vi "calcDemandedPressureOutput.vi"(8 "error in (no error)":errorcluster, 9 "loopPeriod":dbl[unit]=5000.0 min=10.0 max=5000.0, 10 "Pressure Valve Opening (%)":dbl=2.0 min=1.0 max=4.0, 11 "SystemController in":refnum<class "SystemController.lvclass">) -> (0 "error out":errorcluster, 2 "rampOutput (%)":dbl=5000.0 min=10.0 max=5000.0, 3 "SystemController out":refnum<class "SystemController.lvclass">)   [LabVIEW 2015, in "SystemController.lvclass"]
uses:
  SystemController.lvclass
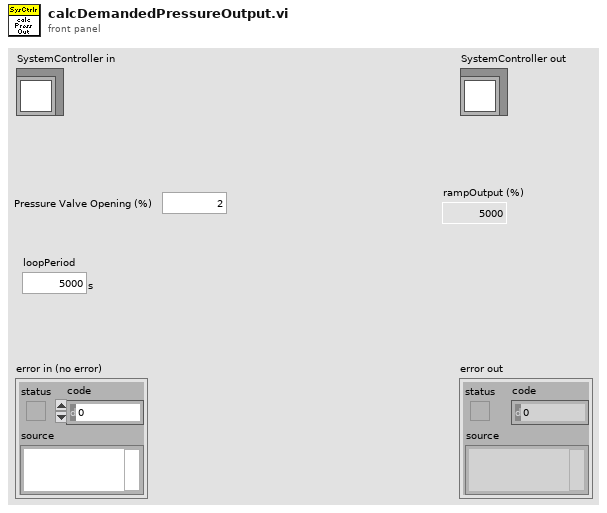
[diagram p1: front panel]
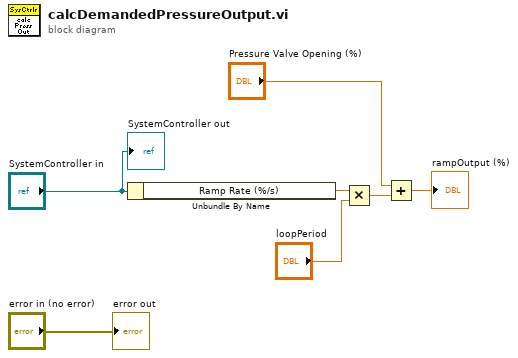
[diagram p0: block diagram]
diagram:
  n1 = Unbundle By Name("SystemController in") -> ("Ramp Rate (%/s)"=w5:dbl[unit])
  n2 = Multiply(x=w5, y="loopPeriod") -> (x*y=w3:dbl)
  n3 = Add(x="Pressure Valve Opening (%)", y=w3) -> (x+y=→"rampOutput (%)":dbl)
  "error out" <- "error in (no error)"
  "SystemController out" <- "SystemController in"
